vi "Cleanup.vi"(8 "error in":errorcluster, 11 "Refnum In":refnum<vi>) -> (0 "error out":errorcluster, 3 "Refnum Out":refnum<vi>)   [LabVIEW 2020, in "SerialCommunicationTransport.lvlib"]
doc: "Cleans up the selected serial comport as the transport method"
uses:
  SerialCommunicationTransport.lvlib
  FirmataClient.lvlib
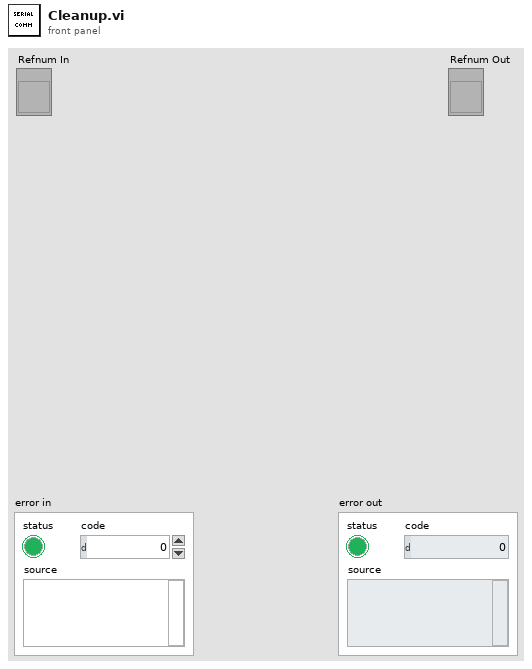
[diagram p1: front panel]
types:
  T1 = typedef "FirmataClient.lvlib/Parameters.ctl" = cluster{"Transport Parameters":T2, "Board Capabilities":map{i32, T4}}
  T2 = typedef "FirmataClient.lvlib/TransportParameters.ctl" = cluster{"Serial Communication":cluster{"Comport":refnum<visa-resource-name>, "No Response Timeout Ms":u32, "Response Complete Timeout Ms":u32, "Max Rx Length":u32, "Baud Rate":u32}, "Selected Transport":T3, "Initializer File Path":path, "Cleaner File Path":path, "Transporter File Path":path}
  T3 = typedef "FirmataClient.lvlib/SupportedTransports.ctl" = enum16{"Serial Communication Port"}
  T4 = typedef "FirmataClient.lvlib/FirmataPinCapabilitiesAndAnalogMapping.ctl" = cluster{"Supported Modes":T5[], "Analog Channel":u8, "Pin Name":string}
  T5 = typedef "FirmataClient.lvlib/FirmataPinCapability.ctl" = cluster{"PinMode":T6, "Resolution":u8}
  T6 = typedef "FirmataClient.lvlib/FirmataPinModes.ctl" = enum16{"DigitalInput", "DigitalOutput", "AnalogInput", "PWM", "Servo", "Shift", "I2C", "OneWire", "Stepper", "Encoder", "Serial", "InputPullup", "Extended.SPI", "Extended.Sonar", "Extended.Tone", "Extended.DHT"}
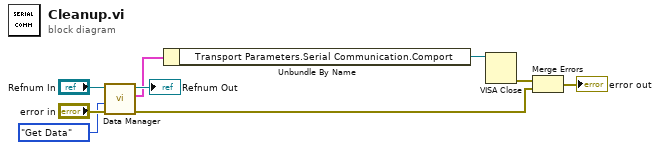
[diagram p0: block diagram]
diagram:
  n1 = call "Data Manager.vi"("error in (no error)"="error in", "Mode"=enum16{"Store Data", "Get Data", "Cleanup"}."Get Data", "Refnum In"="Refnum In") -> ("error out"=w7:errorcluster, "Data Out"=w3:T1, "Refnum Out"=→"Refnum Out":refnum<vi>)  [unwired: 6 in]
  n2 = Unbundle By Name(w3) -> ("Transport Parameters.Serial Communication.Comport"=w2:refnum<visa-resource-name>)
  n3 = VISA Close(VISA resource name=w2) -> (error out=w1:errorcluster)  [unwired: 1 in]
  n4 = Merge Errors(w1, w7) -> (→"error out":errorcluster)
